vi "_2Data_Types.vi"() -> ()   [LabVIEW 2018]
panel:
  out "Boolean 2":bool
  in  "Boolean":bool
  out "String_2":string
  in  "String_1":string
  in  "Float_1":dbl
  out "Float_2":dbl
  in  "Integer_1":dbl
  out "Integer_2":dbl
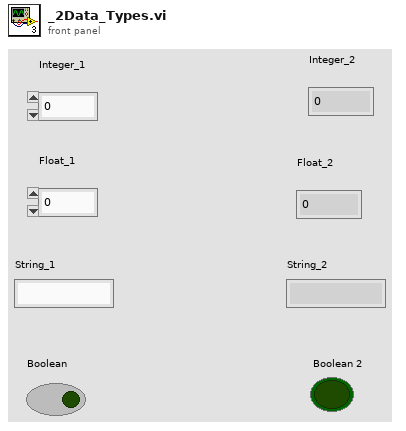
[diagram p1: front panel]
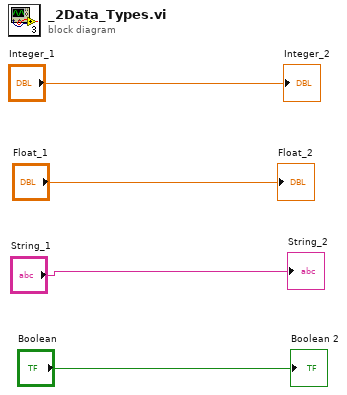
[diagram p0: block diagram]
diagram:
  "Integer_2" <- "Integer_1"
  "Float_2" <- "Float_1"
  "String_2" <- "String_1"
  "Boolean 2" <- "Boolean"
